vi "Step.vi"(8 "error in (no error)":errorcluster, 10 "step size(s)":dbl=30.0 min=0.01, 11 "ODESimulator_LinearConveyor in":refnum<class "ODESimulator_LinearConveyor.lvclass">) -> (0 "error out":errorcluster, 3 "ODESimulator_LinearConveyor out":refnum<class "ODESimulator_LinearConveyor.lvclass">)   [LabVIEW 2017, in "NI_Robotics_Simulator.lvlib" / "ODESimulator_LinearConveyor.lvclass"]
uses:
  <vilib>/robotics/Simulator/Robot Factory/Conveyor/Linear/ODESimulator_LinearConveyor.lvclass
  <vilib>/robotics/Simulator/Robot Factory/Conveyor/Linear/ODESimulator_LinearConveyor.lvclass/ODESimulator_LinearConveyor.ctl
  <vilib>/robotics/Simulator/Robot Factory/Conveyor/Base/ODESimulator_Base_Conveyor.lvclass
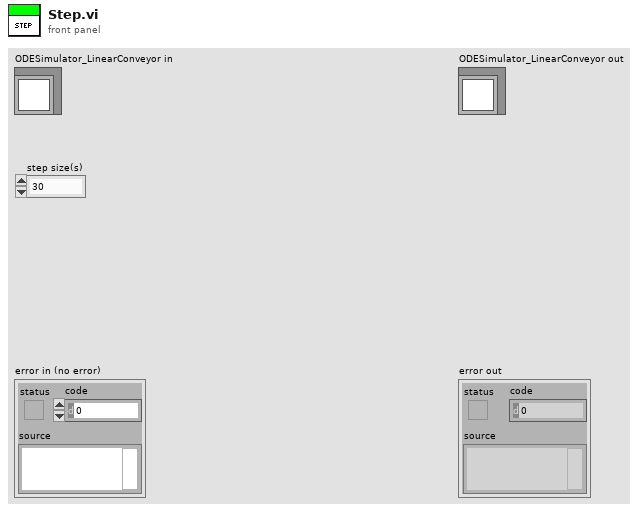
[diagram p1: front panel]
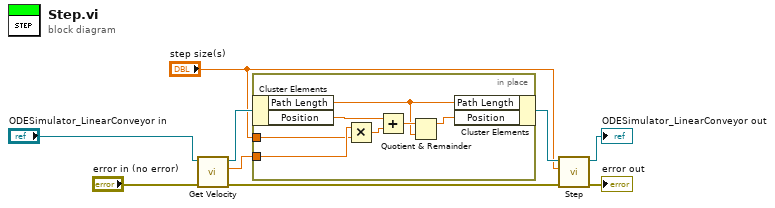
[diagram p0: block diagram]
diagram:
  n1 = call-dynamic "Get Velocity.vi"("error in (no error)"="error in (no error)", "ODESimulator_Base_Conveyor in"="ODESimulator_LinearConveyor in") -> ("error out"=w3:errorcluster, "Velocity"=w2:dbl, "ODESimulator_Base_Conveyor out"=w5:refnum<class "ODESimulator_LinearConveyor.lvclass">)  [unwired: 7 in]
  n2 = in-place {
    in-place-border: w2 -> [w16]
    in-place-border: "step size(s)" -> [w15]
    n3 = in-place-cluster #1(w5) -> ("Path Length"=w11:dbl, "Position"=w13:dbl)
    n4 = Multiply(x=w16, y=w15) -> (x*y=w14:dbl)
    n5 = Add(x=w13, y=w14) -> (x+y=w12:dbl)
    n6 = Quotient & Remainder(x=w12, y=w11) -> (x-y*floor(x/y)=w10:dbl)  [unwired: 1 out]
    n7 = in-place-cluster #1("Path Length"=w11, "Position"=w10) -> (w7:refnum<class "ODESimulator_LinearConveyor.lvclass">)
  }
  n8 = call-parent "Step.vi"("error in (no error)"=w3, "step size(s)"="step size(s)", "3D_Physics_Base in"=w7) -> ("error out"=→"error out":errorcluster, "3D_Physics_Base out"=→"ODESimulator_LinearConveyor out":refnum<class "ODESimulator_LinearConveyor.lvclass">)  [unwired: 7 in]
